vi "CreateVirtualChannelsFromAssets.vi"(8 "error in (no error)":errorcluster, 10 "Channels":T12[](array[typedef]), 11 "AssetNodes":T1[](array[typedef])) -> (0 "error out":errorcluster, 3 "new virtual channels":T12[](array[typedef]))   [LabVIEW 2017, in "McsaVirtualChannel.lvlib"]
uses:
  <vilib>/addons/InsightCM/Devices/Shared/Mcsa/McsaVirtualChannel/McsaVirtualChannel.lvlib
  <vilib>/addons/InsightCM/MessageBus/Base/controls/R2_Channel.ctl
  <vilib>/addons/InsightCM/MessageBus/Base/controls/KeyValuePair.ctl
  <vilib>/addons/InsightCM/MessageBus/Base/controls/Metric.ctl
  <vilib>/addons/InsightCM/MessageBus/Base/controls/AssetNode.ctl
  <vilib>/addons/InsightCM/MessageBus/Base/controls/AssetState.ctl
  <vilib>/addons/InsightCM/MessageBus/Base/controls/OperatingState.ctl
  <vilib>/addons/InsightCM/MessageBus/Base/controls/Trigger.ctl
  <vilib>/addons/InsightCM/MessageBus/Base/controls/Condition.ctl
  <vilib>/addons/InsightCM/MessageBus/Base/controls/TrendAlarmRule.ctl
  <vilib>/addons/InsightCM/MessageBus/Base/controls/TrendAlarmLevel.ctl
  <vilib>/addons/InsightCM/MessageBus/Base/controls/AlarmAction.ctl
  <vilib>/addons/InsightCM/MessageBus/Base/controls/AssetNodeReference.ctl
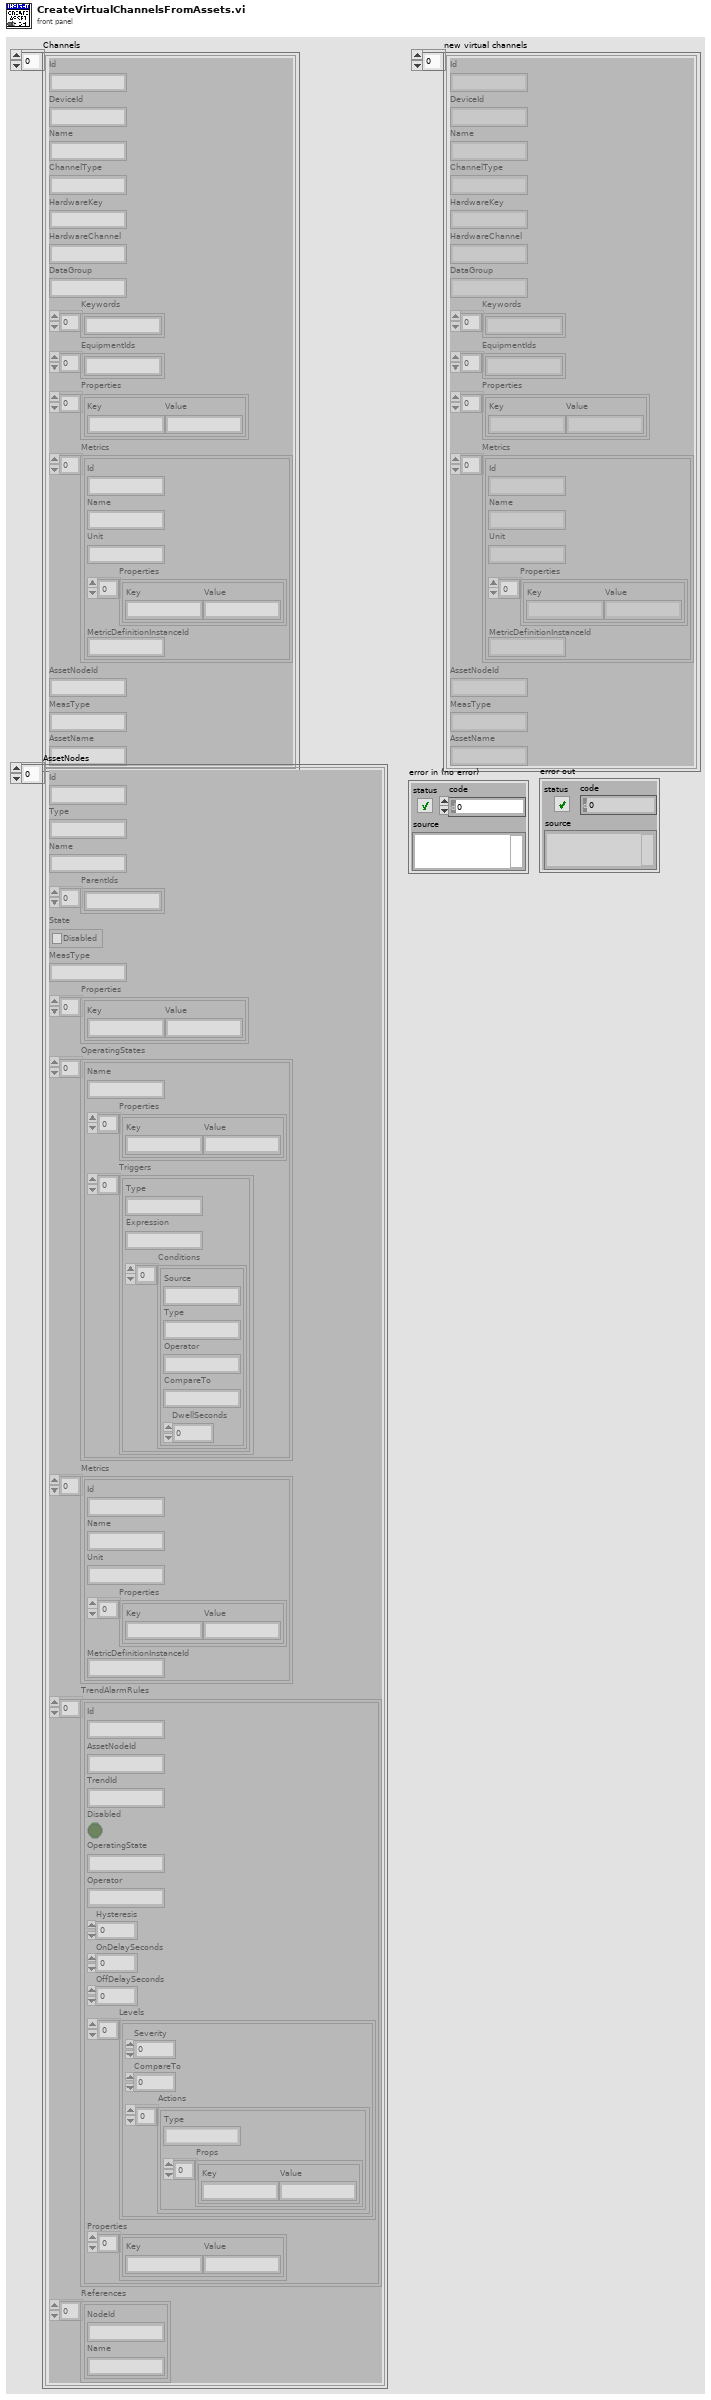
[diagram p1: front panel]
types:
  T1 = typedef "AssetNode.ctl" = cluster{"Id":string, "Type":string, "Name":string, "ParentIds":string[], "State":T2, "MeasType":string, "Properties":T3[], "OperatingStates":T4[], "Metrics":T7[], "TrendAlarmRules":T8[], "References":T11[]}
  T2 = typedef "AssetState.ctl" = cluster{"Disabled":bool}
  T3 = typedef "KeyValuePair.ctl" = cluster{"Key":string, "Value":string}
  T4 = typedef "OperatingState.ctl" = cluster{"Name":string, "Properties":T3[], "Triggers":T5[]}
  T5 = typedef "Trigger.ctl" = cluster{"Type":string, "Expression":string, "Conditions":T6[]}
  T6 = typedef "Condition.ctl" = cluster{"Source":string, "Type":string, "Operator":string, "CompareTo":string, "DwellSeconds":dbl}
  T7 = typedef "Metric.ctl" = cluster{"Id":string, "Name":string, "Unit":string, "Properties":T3[], "MetricDefinitionInstanceId":string}
  T8 = typedef "TrendAlarmRule.ctl" = cluster{"Id":string, "AssetNodeId":string, "TrendId":string, "Disabled":bool, "OperatingState":string, "Operator":string, "Hysteresis":dbl, "OnDelaySeconds":dbl, "OffDelaySeconds":dbl, "Levels":T9[], "Properties":T3[]}
  T9 = typedef "TrendAlarmLevel.ctl" = cluster{"Severity":i32, "CompareTo":dbl, "Actions":T10[]}
  T10 = typedef "AlarmAction.ctl" = cluster{"Type":string, "Props":T3[]}
  T11 = typedef "AssetNodeReference.ctl" = cluster{"NodeId":string, "Name":string}
  T12 = typedef "R2_Channel.ctl" = cluster{"Id":string, "DeviceId":string, "Name":string, "ChannelType":string, "HardwareKey":string, "HardwareChannel":string, "DataGroup":string, "Keywords":string[], "EquipmentIds":string[], "Properties":T3[], "Metrics":T7[], "AssetNodeId":string, "MeasType":string, "AssetName":string}
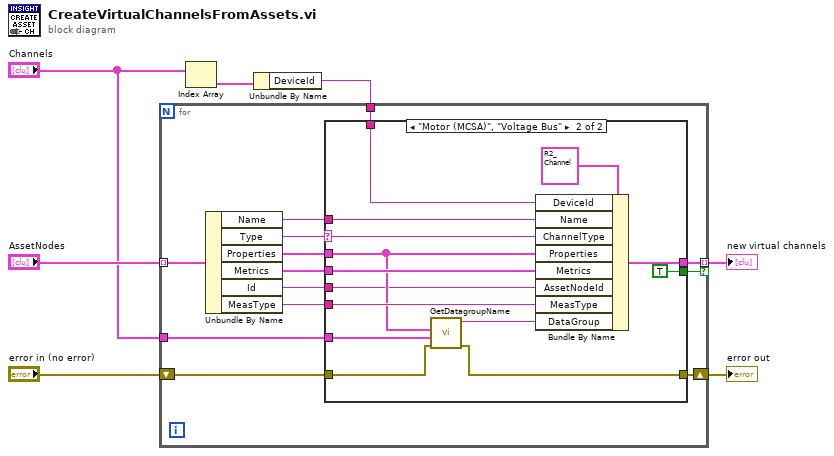
[diagram p0: block diagram]
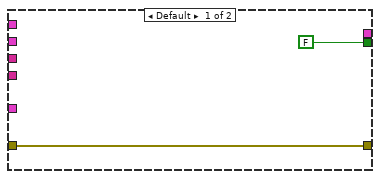
[diagram p2: hidden frame]
diagram:
  n1 = Index Array(array="Channels") -> (element=w5:T12)  [unwired: 1 in]
  n2 = Unbundle By Name(w5) -> ("DeviceId"=w6:string)
  n3 = for {
    tunnel: "AssetNodes" -> [w20] mode=indexing
    tunnel: w6 -> [w19]
    tunnel: [w13] -> w7 mode=indexing if=w11
    tunnel: "Channels" -> [w10]
    shift-right: [w8] -> w1
    shift-left: "error in (no error)" -> [w9]
    n4 = Unbundle By Name(w20) -> ("Name"=w18:string, "Type"=w12:string, "Properties"=w17:T3[], "Metrics"=w16:T7[], "Id"=w15:string, "MeasType"=w14:string)
    n5 = case shown="\"Motor (MCSA)\", \"Voltage Bus\"" w12 {
      selector: w12 -> [_ w31]
      tunnel: w19 -> [_ w36]
      tunnel: w18 -> [_ w35]
      tunnel: w17 -> [_ w29]
      tunnel: w16 -> [_ w34]
      tunnel: w15 -> [_ w26]
      tunnel: w14 -> [_ w33]
      tunnel: [_ w32] -> w13
      tunnel: [FALSE TRUE] -> w11
      tunnel: w10 -> [_ w28]
      tunnel: w9 -> [w21 w25]
      tunnel: [w21 w24] -> w8
      frame Default {
      }
      frame "Motor (MCSA)", "Voltage Bus" {
        n6 = call <vilib>:"GetDatagroupName.vi"("error in (no error)"=w25, "Channels"=w28, "Properties"=w29) -> ("error out"=w24:errorcluster, "Data Group Name"=w27:string)  [unwired: 7 in]
        n7 = Bundle By Name(cluster=T12 {"Id"="", "DeviceId"="", "Name"="", "ChannelType"="", "HardwareKey"="", "HardwareChannel"="", "DataGroup"="", "Keywords"=[], "EquipmentIds"=[], "Properties"=[], "Metrics"=[], "AssetNodeId"="", "MeasType"="", "AssetName"=""} ("Channel"), "DeviceId"=w36, "Name"=w35, "ChannelType"=w31, "Properties"=w29, "Metrics"=w34, "AssetNodeId"=w26, "MeasType"=w33, "DataGroup"=w27) -> (w32:T12)
      }
    }
  }
  "new virtual channels" <- w7
  "error out" <- w1
